vi "transmation.vi"() -> ()   [LabVIEW 2017]
uses:
  <vilib>/addons/Modulation/Digital/General/MT Generate Bits (Galois, PN Order).vi
  <vilib>/addons/Modulation/Digital/Support/Common/Validators/mod_Generate Bits Validate.vi
  <vilib>/addons/Modulation/Analog/support/mod_Set Error Source.vi
  <vilib>/addons/Modulation/Digital/General/subVIs/mod_Generate Bits PN Sequence.vi
  <vilib>/addons/Modulation/Digital/Support/Common/Validators/mod_Generate Filter Coefficients Validate.vi
  <vilib>/addons/Modulation/Digital/General/subVIs/mod_Generate Filter Coefficients.vi
  <vilib>/addons/Modulation/Digital/General/MT Generate MSK System Parameters.vi
  <instrlib>/niUSRP/niUSRP Write Tx Data (CDB Cluster).vi
  <vilib>/addons/Modulation/niDMT.lvlib
panel:
  in  "Boolean":bool
  out "coerced gain":dbl format="%#_6f"
  out "coerced carrier frequency":dbl=100000.0 format="%#_6p"
  out "coerced IQ rate":dbl=100000.0 format="%#_6p"
  in  "active antenna":string
  in  "filter length (symbols)":i32=8
  out "inputSeq":dbl[](graph)
  out "modulation constaltion":T1(graph)
  out "modulation":dbl[](graph)
  out "filter shape":dbl[](graph)
  in  "while loop":bool
  out "error out":errorcluster
  in  "error in (no error)":errorcluster
  in  "gain":dbl format="%#_6f"
  in  "carrier frequency":dbl=100000.0 format="%#_6p"
  in  "IQ rate":dbl=100000.0 format="%#_6p"
  in  "device names":refnum<k15>
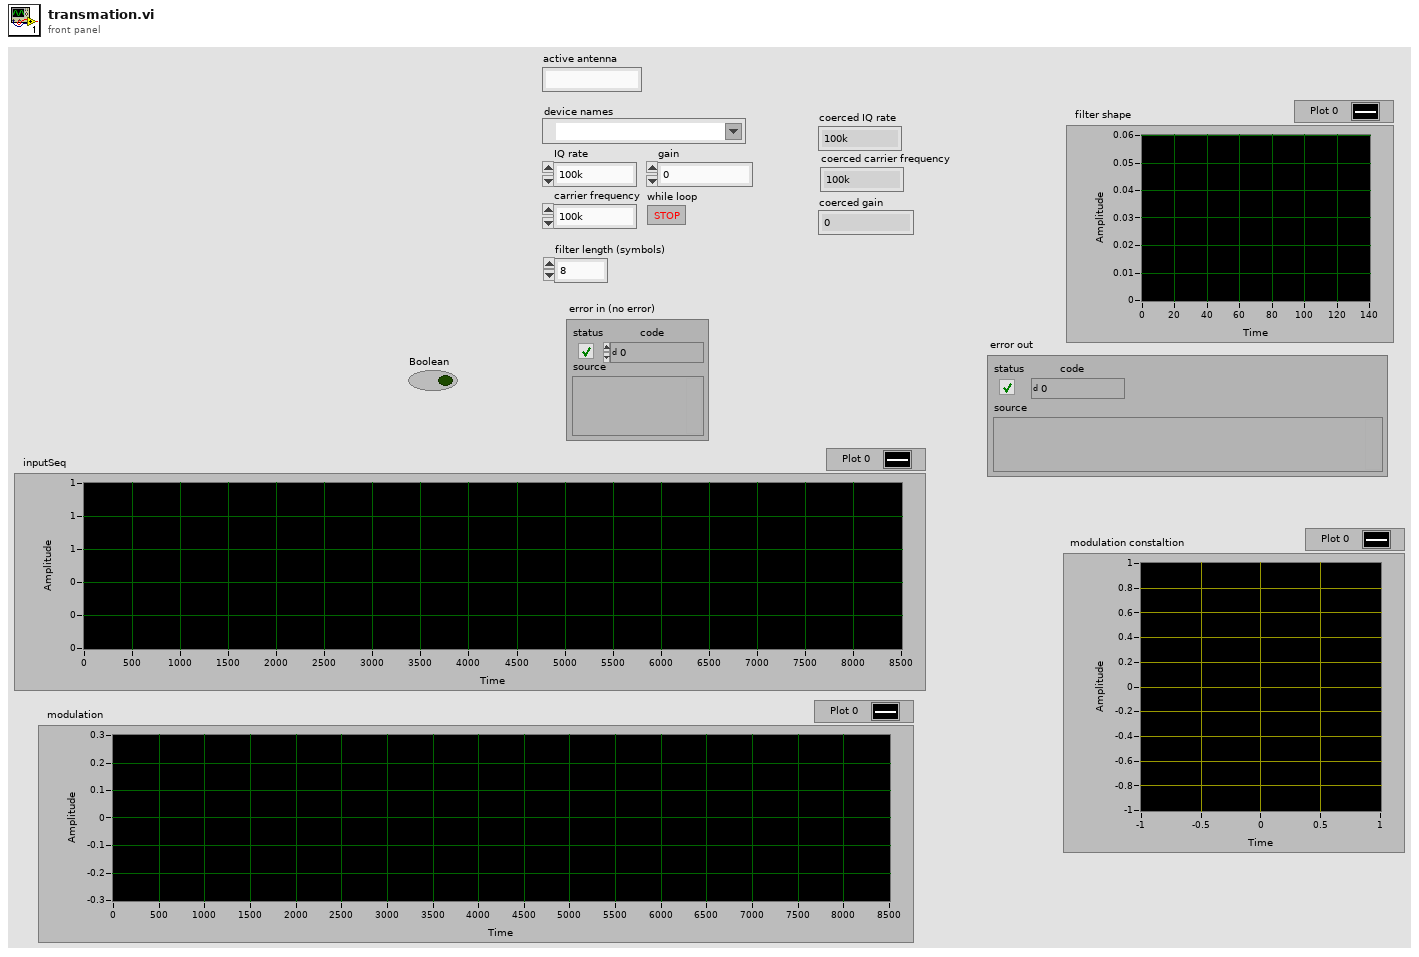
[diagram p1: front panel]
types:
  T1 = cluster{"constellation":dbl[], "oversampled data":dbl[]}[]
  T2 = enum16{"none", "Raised Cosine", "Root Raised Cos", "Gaussian"}
  T3 = enum16{"FSK", "PSK", "QAM", "MSK", "PAM", "ASK", "CPM"}
  T4 = cluster{"differential encoding enable":enum16{"disable", "enable"}, "samples per symbol (16)":i32}
  T5 = typedef "niAMT.lvlib/Complex Data Waveform.ctl" = cluster{"t0":dbl, "dt":dbl, "Y":cdb[]}
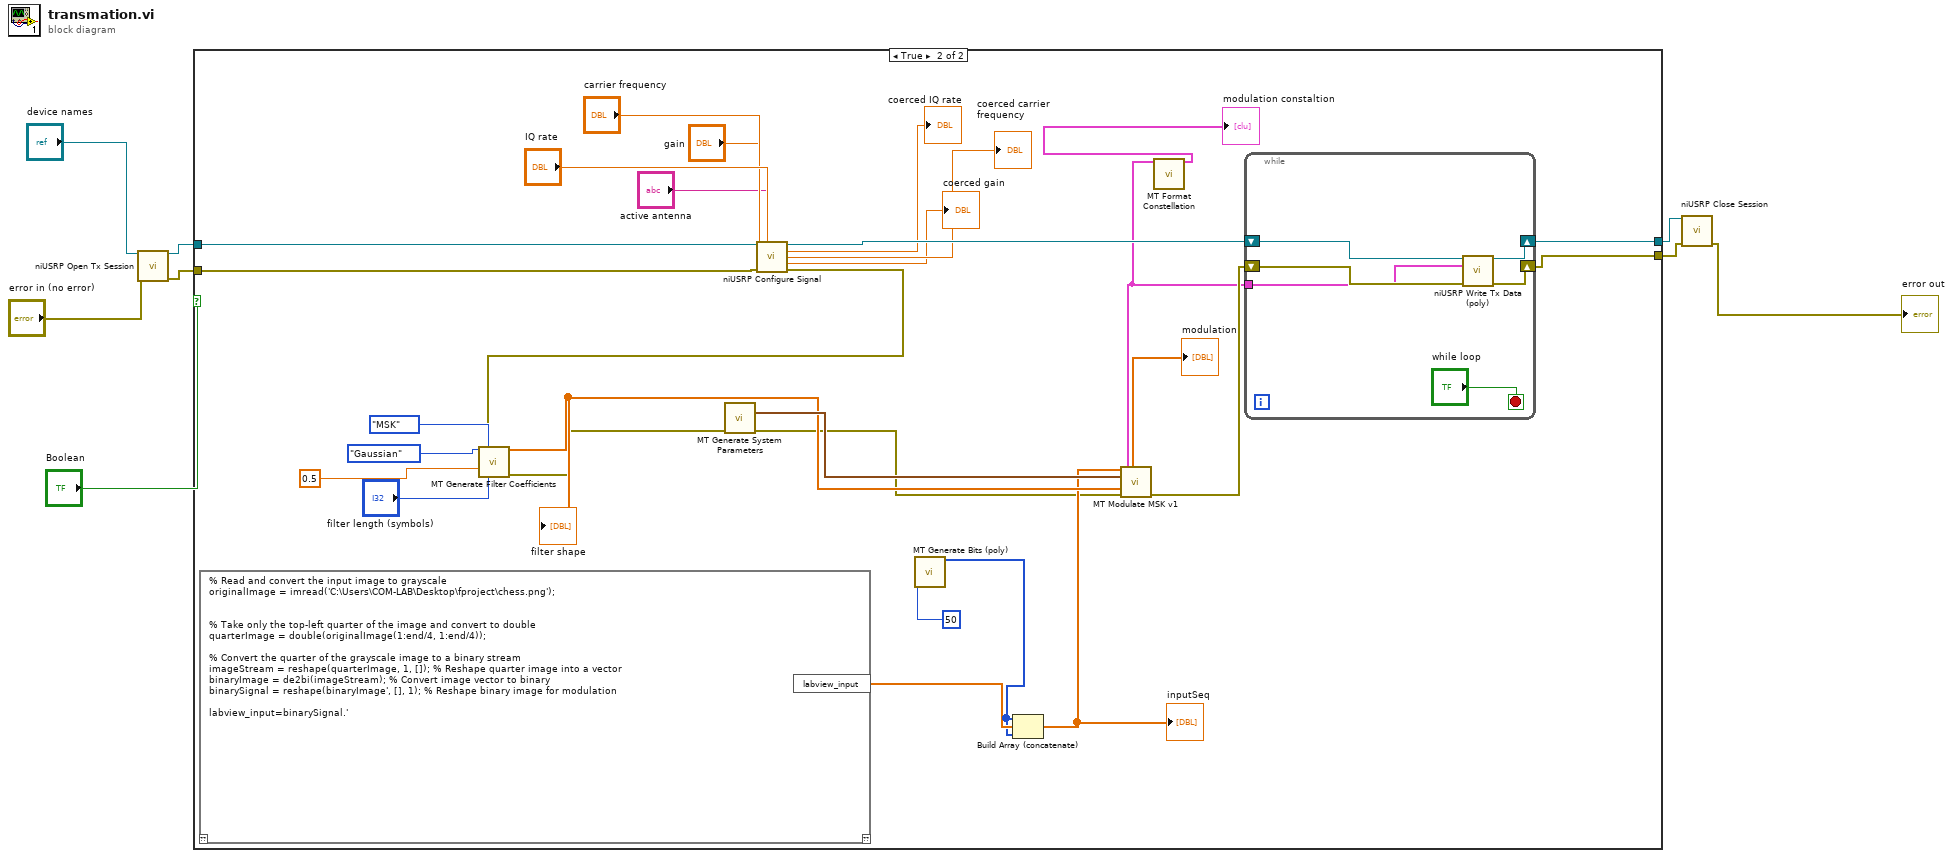
[diagram p0: block diagram]
diagram:
  n1 = call <instrlib>:"niUSRP Open Tx Session.vi"("device names"="device names", "error in (no error)"="error in (no error)") -> ("session handle out"=w5:refnum<k15>, "error out"=w4:errorcluster)  [unwired: 12 in]
  n2 = case shown="True" "Boolean" {
    tunnel: w5 -> [_ w15]
    tunnel: w4 -> [w9 w14]
    tunnel: [w9 w12] -> w3
    tunnel: [_ w13] -> w1
    frame False {
    }
    frame True {
      n3 = script code="% Read and convert the input image to grayscale\noriginalImage = imread('C:\\Users\\COM-LAB\\Desktop\\fproject\\chess.png');\n\n\n% Take only the top-left quarter of the image and convert to double\nquarterImage = double(originalImage(1:end/4, 1:end/4));\n\n% Convert the quarter of the grayscale image to a binary stream\nimageStream = reshape(quarterImage, 1, []); % Reshape quarter image into a vector\nbinaryImage = de2bi(imageStream); % Convert image vector to binary\nbinarySignal = reshape(binaryImage', [], 1); % Reshape binary image for modulation\n\nlabview_input=binarySignal.'"() -> ("labview_input"=w25:dbl[])  [unwired: 1 in, 1 out]
      n4 = call <instrlib>:"niUSRP Configure Signal.vi"("session handle"=w15, "IQ rate"="IQ rate", "carrier frequency"="carrier frequency", "gain"="gain", "error in (no error)"=w14, "active antenna"="active antenna") -> ("session handle out"=w35:refnum<k15>, "coerced IQ rate"=→"coerced IQ rate":dbl, "coerced carrier frequency"=→"coerced carrier frequency":dbl, "coerced gain"=→"coerced gain":dbl, "error out"=w24:errorcluster)  [unwired: 5 in]
      n5 = call <vilib>:"MT Generate Filter Coefficients.vi"("pulse shaping filter (none)"=T2."Gaussian", "modulation type"=T3."MSK", "filter parameter"=0.5, "error in (no error)"=w24, "filter length (symbols)"="filter length (symbols)") -> ("pulse shaping filter coefficients"=w30:dbl[], "error out"=w23:errorcluster)  [unwired: 8 in, 1 out]
      "filter shape" <- w30
      n6 = call-poly <vilib>:"MT Generate System Parameters.vi"("error in (no error)"=w23) -> ("MSK system parameters"=w31:T4, "error out"=w22:errorcluster)  [unwired: 12 in, 1 out]
      n7 = call-poly <vilib>:"MT Generate Bits (poly).vi"("total bits (128)"=50) -> ("output bit stream"=w10:i8[])  [unwired: 12 in, 2 out]
      n8 = Build Array (concatenate)(w10, w25, w10) -> (w29:dbl[])
      "inputSeq" <- w29
      n9 = call <vilib>:"MT Modulate MSK v1.vi"("input bit stream"=w29, "MSK system parameters"=w31, "pulse shaping filter coefficients"=w30, "error in (no error)"=w22) -> ("output complex waveform"=w16:T5, "symbols out"=→"modulation":dbl[], "error out"=w21:errorcluster)  [unwired: 9 in]
      n10 = call <vilib>:"MT Format Constellation.vi"("waveform"=w16) -> ("constellation graph"=→"modulation constaltion":T1)  [unwired: 13 in, 1 out]
      n11 = while {
        shift-right: [w39] -> w12
        shift-left: w21 -> [w44]
        shift-right: [w40] -> w13
        shift-left: w35 -> [w43]
        tunnel: w16 -> [w41]
        stop <- "while loop" stop-if-true
        n12 = call-poly <instrlib>:"niUSRP Write Tx Data (poly).vi"("session handle"=w43, "data"=w41, "error in (no error)"=w44) -> ("session handle out"=w40:refnum<k15>, "error out"=w39:errorcluster)  [unwired: 11 in]
      }
    }
  }
  n13 = call <instrlib>:"niUSRP Close Session.vi"("session handle"=w1, "error in (no error)"=w3) -> ("error out"=→"error out":errorcluster)  [unwired: 13 in]
